vi "create.vi"(8 "error in (no error)":errorcluster, 11 "comic_class in":refnum<class "comic_class.lvclass">) -> (0 "error out":errorcluster, 3 "comic_class out":refnum<class "comic_class.lvclass">)   [LabVIEW 2024, in "comic_class.lvclass"]
uses:
  comic_class.lvclass
  comic_class.lvclass/comic_class.ctl
  <vilib>/httpClient/LabVIEWHTTPClient.lvlib
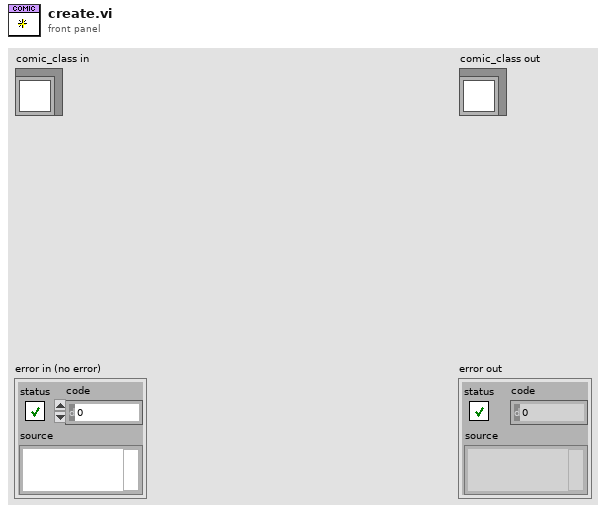
[diagram p1: front panel]
types:
  T1 = typedef "LabVIEWHTTPClient.lvlib/ClientHandle.ctl" = refnum<k1>
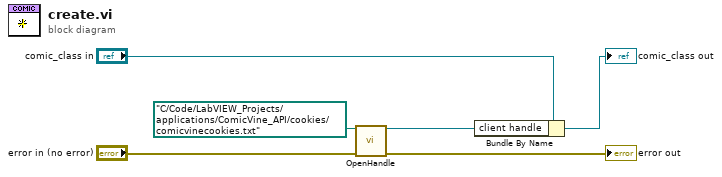
[diagram p0: block diagram]
diagram:
  n1 = call <vilib>:"OpenHandle.vi"("cookie file"=path "C:/Code/LabVIEW_Projects/applications/ComicVine_API/cookies/comicvinecookies.txt", "error in (no error)"="error in (no error)") -> ("client handle out"=w1:T1, "error out"=→"error out":errorcluster)  [unwired: 12 in]
  n2 = Bundle By Name(cluster="comic_class in", "client handle"=w1) -> (→"comic_class out":refnum<class "comic_class.lvclass">)
